vi "Init LSM6DS3.vi"(8 "error in (no error)":errorcluster, 11 "Grove 6 Axis Gyro Accel LSM6DS3 in":refnum<class "Grove 6 Axis Gyro Accel LSM6DS3.lvclass">) -> (0 "error out":errorcluster, 3 "Grove 6 Axis Gyro Accel LSM6DS3 out":refnum<class "Grove 6 Axis Gyro Accel LSM6DS3.lvclass">)   [LabVIEW 2020, in "CTI-Peripheral.lvlib" / "Grove 6 Axis Gyro Accel LSM6DS3.lvclass"]
uses:
  Grove 6 Axis Gyro Accel LSM6DS3.lvclass
  Grove 6 Axis Gyro Accel LSM6DS3.lvclass/Grove 6 Axis Gyro Accel LSM6DS3.ctl
  CTI/I2C Connection/I2C Connection.lvclass/I2C Connection.ctl
  CTI/Session/I2C Write Data.vi
  CTI/Session/I2C Read Data.vi
  CTI/I2C Connection/I2C Connection.lvclass
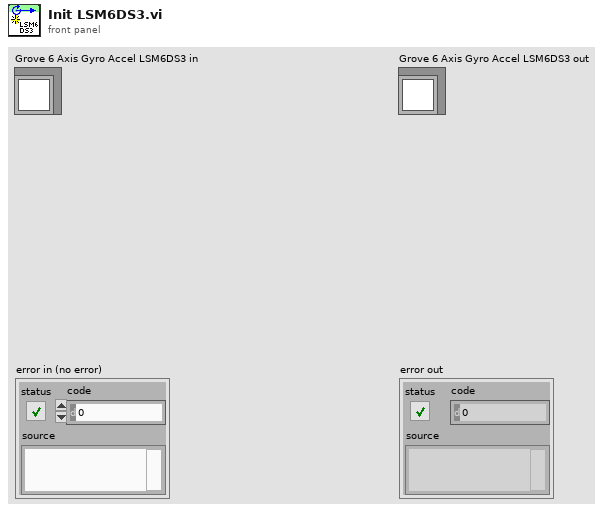
[diagram p1: front panel]
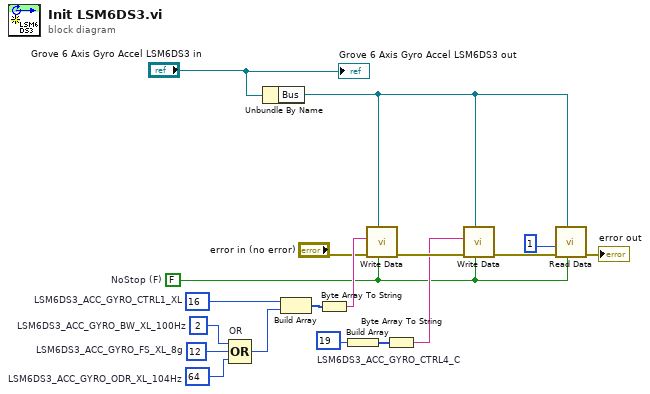
[diagram p0: block diagram]
diagram:
  w11 = u8 19  # LSM6DS3_ACC_GYRO_CTRL4_C
  w13 = u8 64  # LSM6DS3_ACC_GYRO_ODR_XL_104Hz
  w14 = u8 12  # LSM6DS3_ACC_GYRO_FS_XL_8g
  w15 = u8 2  # LSM6DS3_ACC_GYRO_BW_XL_100Hz
  w16 = u8 16  # LSM6DS3_ACC_GYRO_CTRL1_XL
  w1 = FALSE  # NoStop (F)
  n1 = Compound Arithmetic op=OR "OR"(w15, w14, w13) -> (w12:u8)
  n2 = Unbundle By Name("Grove 6 Axis Gyro Accel LSM6DS3 in") -> ("Bus"=w2:refnum<class "I2C Connection.lvclass">)
  n3 = Build Array(w16, w12) -> (w17:u8[])
  n4 = Byte Array To String(unsigned byte array=w17) -> (string=w6:string)
  n5 = Build Array(w11) -> (w10:u8[])
  n6 = call "Write Data.vi"("NoStop (F)"=w1, "I2C Connection"=w2, "error in (no error)"="error in (no error)", "Data"=w6) -> ("error out"=w9:errorcluster)  [unwired: 7 in]
  n7 = Byte Array To String(unsigned byte array=w10) -> (string=w5:string)
  n8 = call "Write Data.vi"("NoStop (F)"=w1, "I2C Connection"=w2, "error in (no error)"=w9, "Data"=w5) -> ("error out"=w8:errorcluster)  [unwired: 7 in]
  n9 = call "Read Data.vi"("NoStop (F)"=w1, "I2C Connection"=w2, "error in (no error)"=w8, "Len"=u8 1) -> ("error out"=→"error out":errorcluster)  [unwired: 6 in, 1 out]
  "Grove 6 Axis Gyro Accel LSM6DS3 out" <- "Grove 6 Axis Gyro Accel LSM6DS3 in"
